vi "Preset PART NUMBER with validation.vi"(8 "error in (no error)":errorcluster, 10 "PART number":string, 11 "VISA resource in":refnum<visa-resource-name>) -> (0 "error out":errorcluster, 3 "VISA resource out":refnum<visa-resource-name>)   [LabVIEW 2025]
uses:
  Preset Number States--enum.ctl
  <instrlib>/Chroma 19052/Chroma 19052.lvlib
panel:
  # "Min 1 char, Max 13 char"
  # "Set PART number"
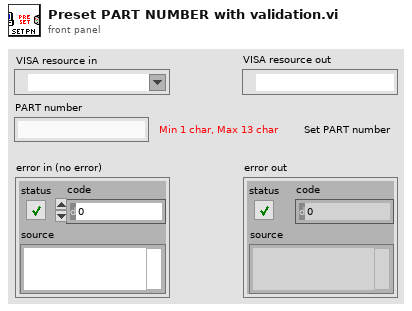
[diagram p1: front panel]
types:
  T1 = typedef "Preset Number States--enum.ctl" = enum16{"Initialize", "Check <=UL", "Check >=LL", "Truncate string", "Send command", "Shutdown"}
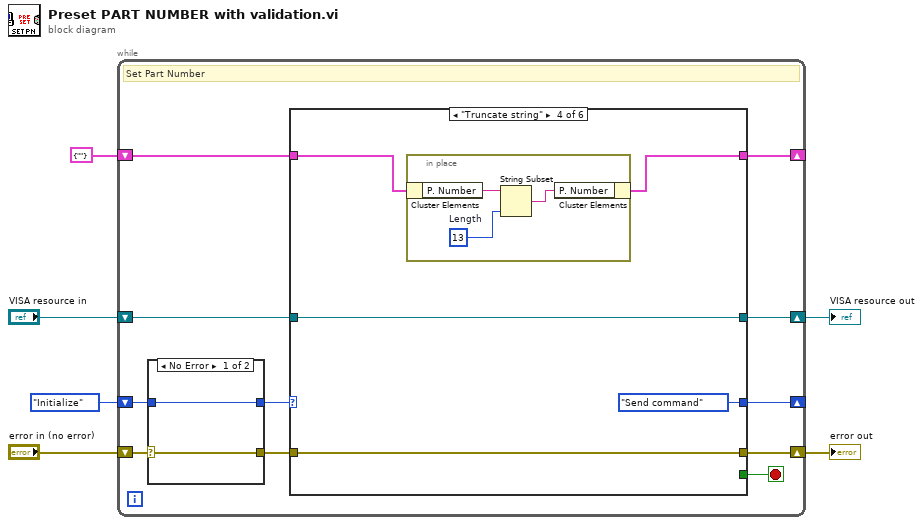
[diagram p0: block diagram]
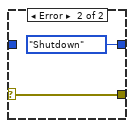
[diagram p2: hidden frame]
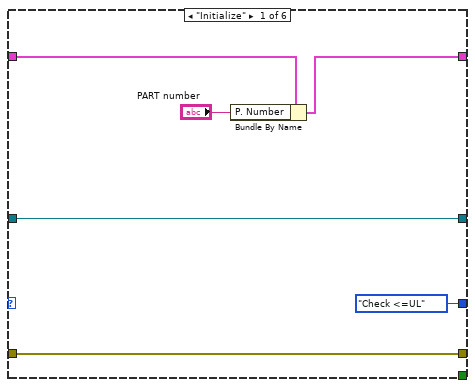
[diagram p3: hidden frame]
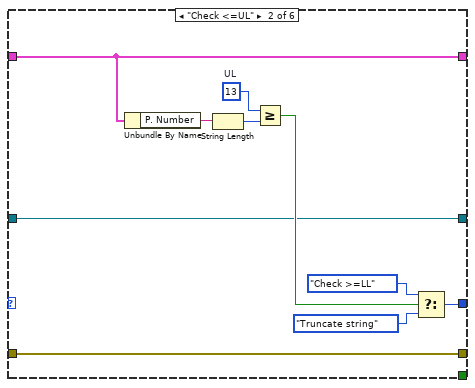
[diagram p4: hidden frame]
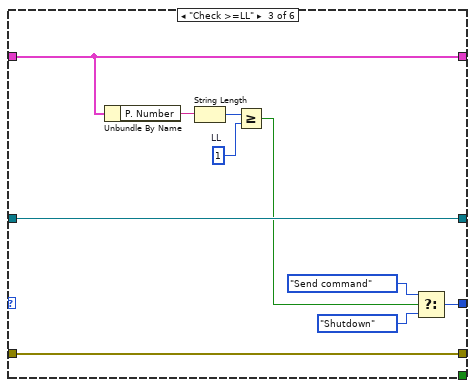
[diagram p5: hidden frame]
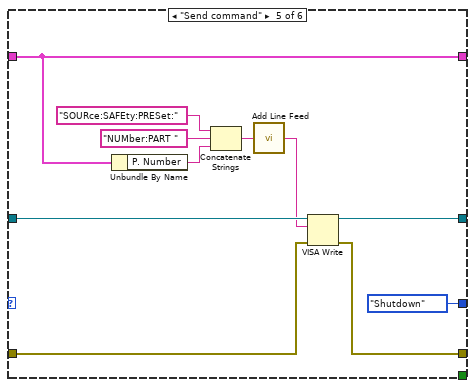
[diagram p6: hidden frame]
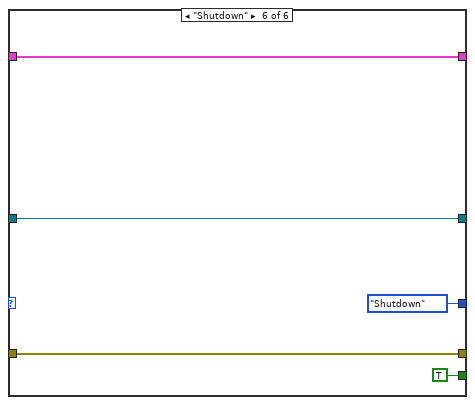
[diagram p7: hidden frame]
diagram:
  n1 = while {
    shift-right: [w15] -> _
    shift-left: Preset_Number_States--enum."Initialize" -> [w14]
    shift-right: [w10] -> w3
    shift-left: "VISA resource in" -> [w13]
    shift-right: [w8] -> _
    shift-left: cluster{"P. Number":string} {"P. Number"=""} -> [w7]
    shift-right: [w11] -> w4
    shift-left: "error in (no error)" -> [w16]
    stop <- w9 stop-if-true
    # "Set Part Number"
    n2 = case shown="No Error" w16 {
      selector: w16 -> [w19 w21]
      tunnel: [w19 w21] -> w12
      tunnel: [w18 Preset_Number_States--enum."Shutdown"] -> w17
      tunnel: w14 -> [w18 _]
      frame No Error {
      }
      frame Error {
      }
    }
    n3 = case shown="\"Truncate string\"" w17 {
      tunnel: [Preset_Number_States--enum."Check <=UL" w34 w43 Preset_Number_States--enum."Send command" Preset_Number_States--enum."Shutdown" Preset_Number_States--enum."Shutdown"] -> w15
      tunnel: w13 -> [w26 w33 w47 w52 w66 w71]
      tunnel: w12 -> [w27 w32 w46 w51 w65 w70]
      tunnel: [w27 w32 w46 w51 w64 w70] -> w11
      tunnel: [w26 w33 w47 w52 w63 w71] -> w10
      tunnel: [_ _ _ _ _ TRUE] -> w9
      tunnel: w7 -> [w25 w31 w40 w49 w56 w67]
      tunnel: [w24 w31 w40 w48 w56 w67] -> w8
      frame "Initialize" {
        n4 = Bundle By Name(cluster=w25, "P. Number"="PART number") -> (w24:cluster{"P. Number":string})
      }
      frame "Check <=UL" {
        w37 = 13  # UL
        n5 = Unbundle By Name(w31) -> ("P. Number"=w30:string)
        n6 = String Length(string=w30) -> (length=w36:i32)
        n7 = Greater Or Equal?(x=w37, y=w36) -> (x >= y?=w35:bool)
        n8 = Select(t=Preset_Number_States--enum."Check >=LL", s=w35, f=Preset_Number_States--enum."Truncate string") -> (s? t:f=w34:T1)
      }
      frame "Check >=LL" {
        w44 = 1  # LL
        n9 = Unbundle By Name(w40) -> ("P. Number"=w39:string)
        n10 = String Length(string=w39) -> (length=w45:i32)
        n11 = Greater Or Equal?(x=w45, y=w44) -> (x >= y?=w42:bool)
        n12 = Select(t=Preset_Number_States--enum."Send command", s=w42, f=Preset_Number_States--enum."Shutdown") -> (s? t:f=w43:T1)
      }
      frame "Truncate string" {
        n13 = in-place "In Place Element Structure" {
          w55 = 13  # Length
          n14 = in-place-cluster #1 ("Unbundle / Bundle Elements")(w49) -> ("P. Number"=w54:string)
          n15 = String Subset(string=w54, length (rest)=w55) -> (substring=w53:string)  [unwired: 1 in]
          n16 = in-place-cluster #1 ("Unbundle / Bundle Elements")("P. Number"=w53) -> (w48:cluster{"P. Number":string})
        }
      }
      frame "Send command" {
        n17 = Unbundle By Name(w56) -> ("P. Number"=w59:string)
        n18 = Concatenate Strings("SOURce:SAFEty:PRESet:", "NUMber:PART ", w59) -> (w58:string)
        n19 = call <instrlib>:"Add Line Feed.vi"("Command string"=w58) -> ("Concatenated string"=w57:string)  [unwired: 4 in]
        n20 = VISA Write(VISA resource name=w66, write buffer=w57, error in (no error)=w65) -> (VISA resource name out=w63:refnum<visa-resource-name>, error out=w64:errorcluster)  [unwired: 1 out]
      }
      frame "Shutdown" {
      }
    }
  }
  "error out" <- w4
  "VISA resource out" <- w3
